vi "CRYGet CurveNames From Analysis.vi"(4 "Spectral Scaling":u16, 6 "Unit Info":T2={"Y unit In"="dB", "dB ref In"=1.0, "Y unit Out"="dB", "dB ref Out"=1.0, "Y unit Curve"="dB", "dB ref Curve"=1.0, "Y data  Curve"=0, "Y data Time"=0}, 8 "Harmonics array In":dbl[](array[numeric]) format="%.2f", 9 "Additional Option":T4(ring), 10 "Select Option":T5(ring), 11 "Algorithm":T6(ring)) -> (0 "Unit Info Out":T1, 1 "Display":T3={"display X"=TRUE, "display Y"=TRUE, "display Z"=TRUE}, 2 "Result":bool, 3 "Curves Name Out":string[](array[string]))   [LabVIEW 2013]
uses:
  Typedef Control/CRYUnit Info Cluster.ctl
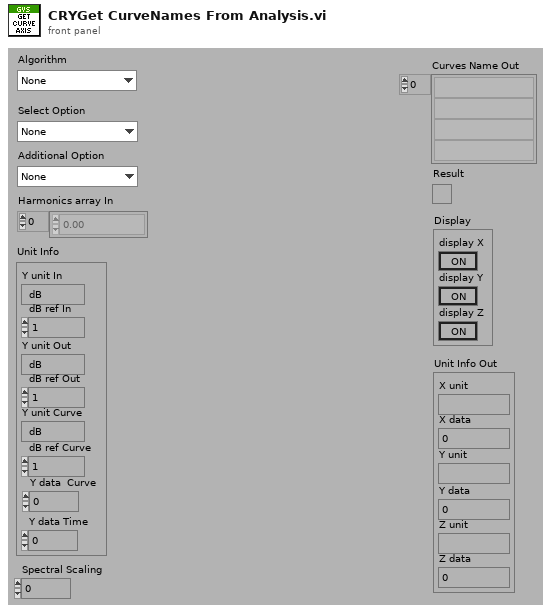
[diagram p1: front panel]
types:
  T1 = cluster{"X unit":string, "X data":u16, "Y unit":string, "Y data":u16, "Z unit":string, "Z data":u16}
  T2 = typedef "CRYUnit Info Cluster.ctl" = cluster{"Y unit In":string, "dB ref In":dbl, "Y unit Out":string, "dB ref Out":dbl, "Y unit Curve":string, "dB ref Curve":dbl, "Y data  Curve":u16, "Y data Time":u16}
  T3 = cluster{"display X":bool, "display Y":bool, "display Z":bool}
  T4 = enum16{"None", "Harmonic", "Intermodulation", "Difference", "DC Connect Measurement", "Complex", "Power"}
  T5 = enum16{"None", "Standard Error", "Confidence Limits", "Total Noise", "Harmonics meas.frq.", "Total Distortion", "THD", "THD Normalized", "THD + Noise", "Rub & Buzz", "Rub & Buzz Norm'd", "Total IM", "Total IMD", "Total IMD + Noise", "Total Diff", "Total DFD", "Total DFD + Noise", "Impulse Response", "Deconvolved Response", "Auto-Spectrum(Stimulus)", "Auto-Spectrum(Response)", "Frequency Response", "Cross-Spectrum", "Coherence", "Non-Coherence", "Signal-Noise Ratio", "Coherent Power", "Non-Coherent Power", "Non-Coherent Distortion", "Auto-Correlation(Stimulus)", "Auto-Correlation(Response)", "Cross-Correlation", "Impedence", "Auto Delay", "Time Envelop", "Loose Particle", "A(in Voltage)", "V(in Current)"}
  T6 = enum16{"None", "Broadband RMS", "Spectrum", "Hamonic Track", "Heterodyne", "Time Selective Response", "Multitone", "Transfer Function"}
  T7 = enum16{"None", "Standard Error", "Confidence Limits", "Total Noise", "Harmonics meas.frq.", "Total Distortion", "THD", "THD Normalized", "THD + Noise", "Rub & Buzz", "Rub & Buzz Norm'd", "Total IM", "Total IMD", "Total IMD + Noise", "Total Diff", "Total DFD", "Total DFD + Noise", "Impulse Response", "Deconvolved Response", "Auto-Spectrum(Stimulus)", "Auto-Spectrum(Response)", "Frequency Response", "Cross-Spectrum", "Coherence", "Non-Coherence", "Signal-Noise Ratio", "Coherent Power", "Non-Coherent Power", "Non-Coherent Distortion", "Auto-Correlation(Stimulus)", "Auto-Correlation(Response)", "Cross-Correlation", "Impedence", "Auto Delay", "Time Envelop", "Loose Particle"}
  T8 = cluster{"X unit":string, "X data":u16, "Y unit Curve":string, "Y data  Curve":u16, "Z unit":string, "X data":u16}
  T9 = cluster{"X unit":string, "X data":u16, string, "Y data  Curve":u16, "Z unit":string, "X data":u16}
  T10 = cluster{"X unit":string, "X data":u16, "Y unit Out":string, "Y data  Curve":u16, "Z unit":string, "X data":u16}
  T11 = cluster{"X unit":string, "X data":u16, "X unit":string, "X data":u16, "Z unit":string, "X data":u16}
  T12 = cluster{"X unit":string, "X data":u16, string, "Y data Time":u16, "Z unit":string, "X data":u16}
  T13 = cluster{"X unit":string, "X data":u16, "Y unit In":string, "Y data  Curve":u16, "Z unit":string, "X data":u16}
  T14 = cluster{"X unit":string, "X data":u16, "Z unit":string, "X data":u16, "Z unit":string, "X data":u16}
  T15 = cluster{"X unit":string, "X data":u16, "Y unit Out":string, "Y data Time":u16, "Z unit":string, "X data":u16}
  T16 = cluster{"X unit":string, "X data":u16, "Y unit In":string, "Y data Time":u16, "Z unit":string, "X data":u16}
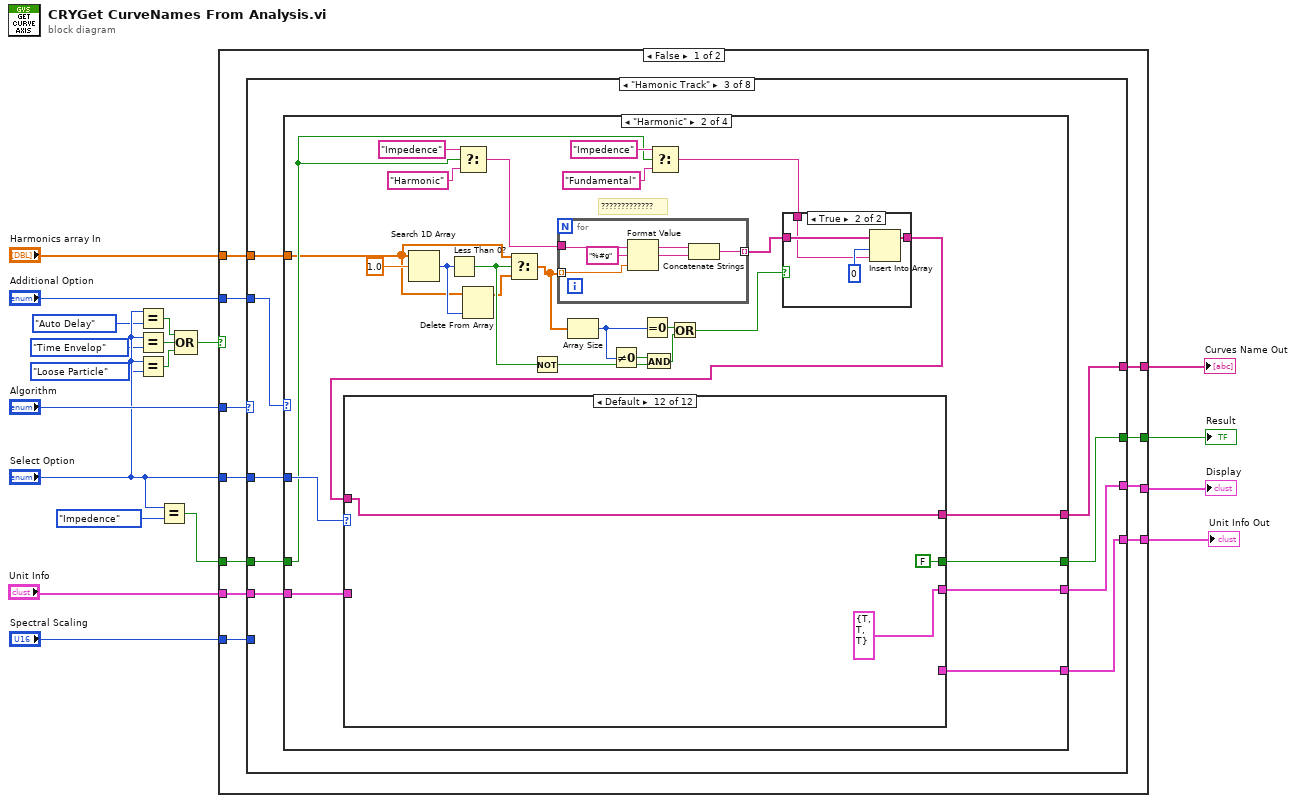
[diagram p0: block diagram]
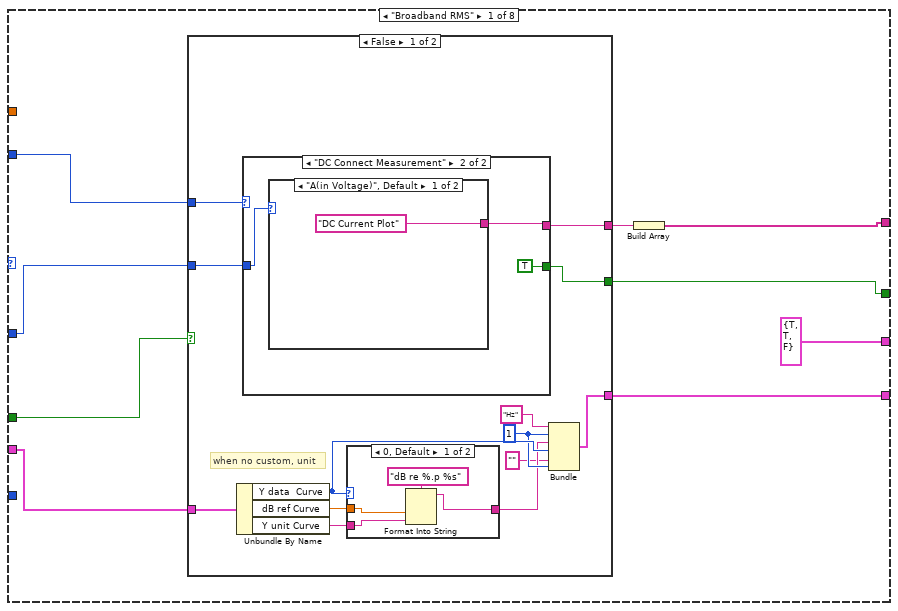
[diagram p2: hidden frame]
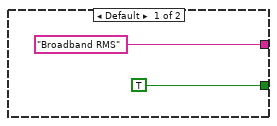
[diagram p4: hidden frame]
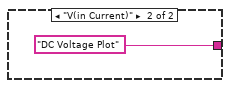
[diagram p5: hidden frame]
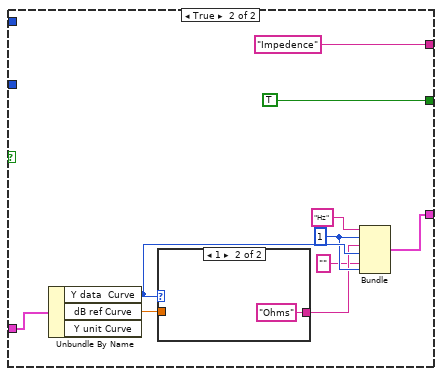
[diagram p6: hidden frame]
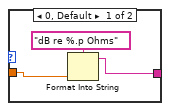
[diagram p7: hidden frame]
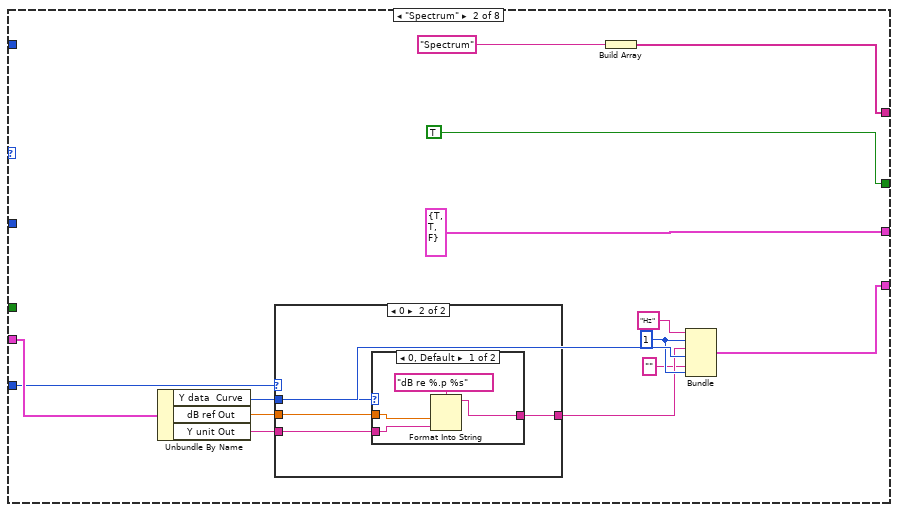
[diagram p8: hidden frame]
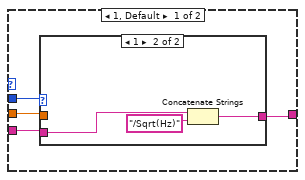
[diagram p9: hidden frame]
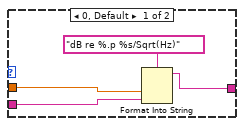
[diagram p10: hidden frame]
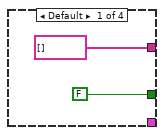
[diagram p12: hidden frame]
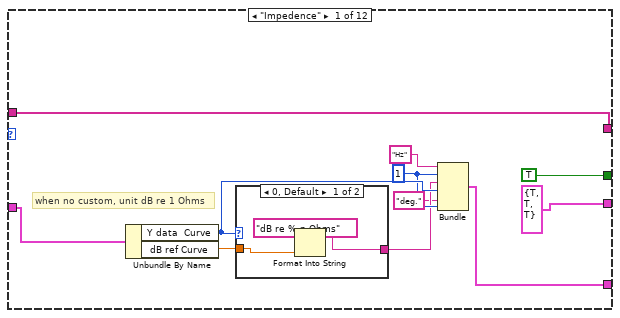
[diagram p14: hidden frame]
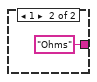
[diagram p15: hidden frame]
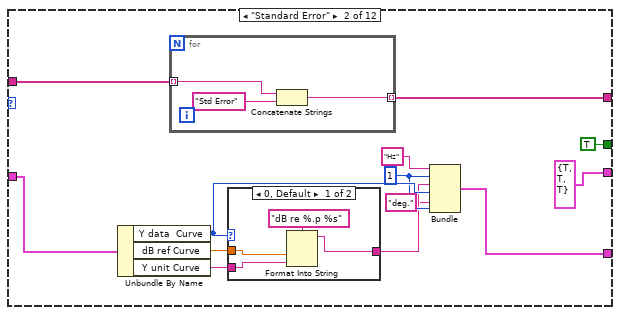
[diagram p16: hidden frame]
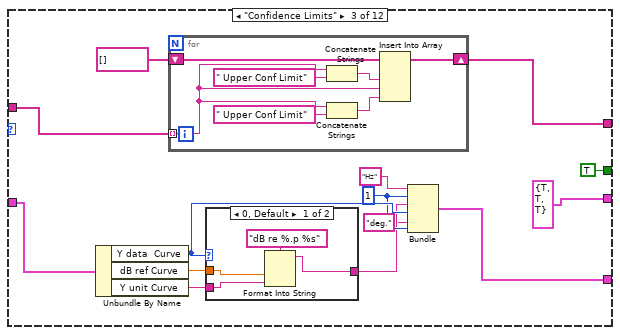
[diagram p18: hidden frame]
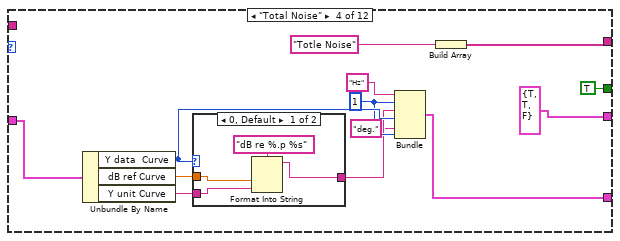
[diagram p20: hidden frame]
diagram:
  n1 = Equal?(x="Select Option", y=T7."Auto Delay") -> (x = y?=w14:bool)
  n2 = Equal?(x="Select Option", y=T7."Time Envelop") -> (x = y?=w13:bool)
  n3 = Equal?(x="Select Option", y=T7."Loose Particle") -> (x = y?=w12:bool)
  n4 = Equal?(x="Select Option", y=T7."Impedence") -> (x = y?=w10:bool)
  n5 = Compound Arithmetic op=OR(w14, w13, w12) -> (w11:bool)
  n6 = case shown="False" w11 {
    tunnel: "Algorithm" -> [w30 _]
    tunnel: "Select Option" -> [w29 w1352]
    tunnel: "Harmonics array In" -> [w28 _]
    tunnel: w10 -> [w27 _]
    tunnel: [w26 w1354] -> w17
    tunnel: [w25 w1353] -> w16
    tunnel: "Additional Option" -> [w24 _]
    tunnel: [w23 w1351] -> w4
    tunnel: "Unit Info" -> [w22 w1349]
    tunnel: [w21 w1350] -> w2
    tunnel: "Spectral Scaling" -> [w20 _]
    frame False {
      n7 = case shown="\"Hamonic Track\"" w30 {
        tunnel: w29 -> [w34 _ w118 _ w667 w777 w1012 _]
        tunnel: w28 -> [_ _ w121 _ w666 _ _ _]
        tunnel: w24 -> [w39 _ w120 _ _ w778 w1011 _]
        tunnel: w27 -> [w35 _ w119 w660 w668 w776 w1010 _]
        tunnel: [w37 w91 w117 w656 w665 w774 w1008 string[] []] -> w25
        tunnel: [w36 TRUE ("Result") w116 TRUE ("Result") w664 w773 w1007 FALSE ("Result")] -> w26
        tunnel: [T3 {"display X"=TRUE, "display Y"=TRUE, "display Z"=FALSE} T3 {"display X"=TRUE, "display Y"=TRUE, "display Z"=FALSE} w115 T3 {"display X"=TRUE, "display Y"=TRUE, "display Z"=TRUE} T3 {"display X"=TRUE, "display Y"=TRUE, "display Z"=TRUE} w772 w1006 _] -> w23
        tunnel: w22 -> [w31 w81 w113 _ w661 w771 w1004 _]
        tunnel: [w32 w80 w114 _ w662 w770 w1005 _] -> w21
        tunnel: w20 -> [_ w79 _ _ _ _ _ _]
        frame "Broadband RMS" {
          n8 = case shown="False" w35 {
            tunnel: [w51 "Impedence" ("string")] -> w38
            tunnel: w39 -> [w52 _]
            tunnel: [w50 TRUE ("Result")] -> w36
            tunnel: w34 -> [w49 _]
            tunnel: [w40 w65] -> w32
            tunnel: w31 -> [w41 w66]
            frame False {
              w45 = u16 1 ("X data")
              # "when no custom, unit"
              n9 = Unbundle By Name(w41) -> ("Y data  Curve"=w48:u16, "dB ref Curve"=w46:dbl, "Y unit Curve"=w47:string)
              n10 = case shown="\"DC Connect Measurement\"" w52 {
                tunnel: ["Broadband RMS" ("f") w62] -> w51
                tunnel: [TRUE ("Result") TRUE ("Result")] -> w50
                tunnel: w49 -> [_ w60]
                frame Default {
                }
                frame "DC Connect Measurement" {
                  n11 = case shown="\"A(in Voltage)\", Default" w60 {
                    tunnel: ["DC Current Plot" ("f") "DC Voltage Plot" ("f")] -> w62
                    frame "A(in Voltage)", Default {
                    }
                    frame "V(in Current)" {
                    }
                  }
                }
              }
              n12 = case shown="0, Default" w48 {
                tunnel: [w53 w57] -> w44
                tunnel: w46 -> [w54 _]
                tunnel: w47 -> [w55 w57]
                frame 0, Default {
                  n13 = Format Into String(format string="dB re %.p %s", w54, w55) -> (resulting string=w53:string)  [unwired: 2 in, 1 out]
                }
                frame 1 {
                }
              }
              n14 = Bundle("X unit"="Hz", "X data"=w45, "Y unit Curve"=w44, "Y data  Curve"=w48, "Z unit"="", "X data"=w45) -> (w40:T8)  [unwired: 1 in]
            }
            frame True {
              w70 = u16 1 ("X data")
              n15 = Unbundle By Name(w66) -> ("Y data  Curve"=w72:u16, "dB ref Curve"=w71:dbl)  [unwired: 1 out]
              n16 = case shown="1" w72 {
                tunnel: [w75 "Ohms"] -> w69
                tunnel: w71 -> [w76 _]
                frame 0, Default {
                  n17 = Format Into String(format string="dB re %.p Ohms", w76) -> (resulting string=w75:string)  [unwired: 2 in, 1 out]
                }
                frame 1 {
                }
              }
              n18 = Bundle("X unit"="Hz", "X data"=w70, w69, "Y data  Curve"=w72, "Z unit"="", "X data"=w70) -> (w65:T9)  [unwired: 1 in]
            }
          }
          n19 = Build Array(w38) -> (w37:string[])
        }
        frame "Spectrum" {
          w85 = u16 1 ("X data")
          n20 = Unbundle By Name(w81) -> ("Y data  Curve"=w88:u16, "dB ref Out"=w86:dbl, "Y unit Out"=w87:string)
          n21 = case shown="0" w79 {
            tunnel: w88 -> [w93 w107]
            tunnel: w87 -> [w95 w106]
            tunnel: w86 -> [w94 w105]
            tunnel: [w96 w104] -> w84
            frame 1, Default {
              n22 = case shown="1" w93 {
                tunnel: [w97 w101] -> w96
                tunnel: w94 -> [w98 _]
                tunnel: w95 -> [w99 w102]
                frame 0, Default {
                  n23 = Format Into String(format string="dB re %.p %s/Sqrt(Hz)", w98, w99) -> (resulting string=w97:string)  [unwired: 2 in, 1 out]
                }
                frame 1 {
                  n24 = Concatenate Strings(w102, "/Sqrt(Hz)" ("Y unit In")) -> (w101:string)
                }
              }
            }
            frame 0 {
              n25 = case shown="0, Default" w107 {
                tunnel: [w108 w112] -> w104
                tunnel: w105 -> [w109 _]
                tunnel: w106 -> [w110 w112]
                frame 0, Default {
                  n26 = Format Into String(format string="dB re %.p %s", w109, w110) -> (resulting string=w108:string)  [unwired: 2 in, 1 out]
                }
                frame 1 {
                }
              }
            }
          }
          n27 = Build Array("Spectrum" ("f")) -> (w91:string[])
          n28 = Bundle("X unit"="Hz", "X data"=w85, "Y unit Out"=w84, "Y data  Curve"=w88, "Z unit"="", "X data"=w85) -> (w80:T10)  [unwired: 1 in]
        }
        frame "Hamonic Track" {
          n29 = case shown="\"Harmonic\"" w120 {
            tunnel: w121 -> [_ w129 w342 w502]
            tunnel: w119 -> [_ w130 w341 w501]
            tunnel: w118 -> [_ w150 w340 w500]
            tunnel: [string[] [] w128 w338 w498] -> w117
            tunnel: [FALSE ("Result") w127 w337 w497] -> w116
            tunnel: [_ w126 w336 w494] -> w115
            tunnel: [_ w125 w335 w495] -> w114
            tunnel: w113 -> [_ w124 w334 w496]
            frame Default {
            }
            frame "Harmonic" {
              # "?????????????"
              n30 = Search 1D Array(1D array=w129, element=1.0) -> (index of element=w139:i32)  [unwired: 1 out]
              n31 = Less Than 0?(x=w139) -> (x < 0?=w146:bool)
              n32 = Select(t="Impedence", s=w130, f="Harmonic" ("string")) -> (s? t:f=w135:string)
              n33 = Delete From Array(array=w129, index=w139) -> (array with subset deleted=w140:dbl[])  [unwired: 1 in, 1 out]
              n34 = Select(t=w129, s=w146, f=w140) -> (s? t:f=w142:dbl[])
              n35 = Not(x=w146) -> (.not. x?=w147:bool)
              n36 = for {
                tunnel: w142 -> [w159] mode=indexing
                tunnel: [w157] -> w141 mode=indexing
                tunnel: w135 -> [w156]
                n37 = Format Value(format string="%#g", value (0)=w159) -> (output string=w158:string)  [unwired: 1 out]
                n38 = Concatenate Strings(w156, w158) -> (w157:string)
              }
              n39 = Array Size(array=w142) -> (size(s)=w144:i32)
              n40 = Not Equal To 0?(x=w144) -> (x != 0?=w145:bool)
              n41 = Equal To 0?(x=w144) -> (x = 0?=w143:bool)
              n42 = And(x=w145, y=w147) -> (x .and. y?=w148:bool)
              n43 = Select(t="Impedence", s=w130, f="Fundamental" ("string")) -> (s? t:f=w132:string)
              n44 = Or(x=w143, y=w148) -> (x .or. y?=w149:bool)
              n45 = case shown="True" w149 {
                tunnel: w141 -> [w151 w154]
                tunnel: [w151 w153] -> w131
                tunnel: w132 -> [_ w152]
                frame False {
                }
                frame True {
                  n46 = Insert Into Array(array=w154, index=0, new element=w152) -> (w153:string[])
                }
              }
              n47 = case shown="Default" w150 {
                tunnel: w131 -> [w171 w188 w209 _ w253 _ _ _ _ _ _ w332]
                tunnel: [w171 w187 w208 w234 w252 w279 w293 w302 w311 w320 w329 w332] -> w128
                tunnel: [TRUE ("Result") TRUE ("Result") TRUE ("Result") TRUE ("Result") TRUE ("Result") TRUE ("Result") TRUE ("Result") TRUE ("Result") TRUE ("Result") TRUE ("Result") TRUE ("Result") FALSE ("Result")] -> w127
                tunnel: [T3 {"display X"=TRUE, "display Y"=TRUE, "display Z"=TRUE} T3 {"display X"=TRUE, "display Y"=TRUE, "display Z"=TRUE} T3 {"display X"=TRUE, "display Y"=TRUE, "display Z"=TRUE} T3 {"display X"=TRUE, "display Y"=TRUE, "display Z"=FALSE} T3 {"display X"=TRUE, "display Y"=TRUE, "display Z"=TRUE} T3 {"display X"=TRUE, "display Y"=TRUE, "display Z"=TRUE} T3 {"display X"=TRUE, "display Y"=TRUE, "display Z"=FALSE} T3 {"display X"=TRUE, "display Y"=TRUE, "display Z"=FALSE} T3 {"display X"=TRUE, "display Y"=TRUE, "display Z"=FALSE} T3 {"display X"=TRUE, "display Y"=TRUE, "display Z"=FALSE} T3 {"display X"=TRUE, "display Y"=TRUE, "display Z"=FALSE} T3 {"display X"=TRUE, "display Y"=TRUE, "display Z"=TRUE}] -> w126
                tunnel: [w161 w177 w198 w224 w242 w269 w286 w295 w304 w313 w322 _] -> w125
                tunnel: w124 -> [w163 w178 w199 w223 w243 w268 _ _ _ _ _ _]
                frame "Impedence" {
                  w166 = u16 1 ("X data")
                  # "when no custom, unit dB re 1 Ohms"
                  n48 = Unbundle By Name(w163) -> ("Y data  Curve"=w168:u16, "dB ref Curve"=w167:dbl)
                  n49 = case shown="0, Default" w168 {
                    tunnel: [w172 "Ohms"] -> w165
                    tunnel: w167 -> [w173 _]
                    frame 0, Default {
                      n50 = Format Into String(format string="dB re %.p Ohms", w173) -> (resulting string=w172:string)  [unwired: 2 in, 1 out]
                    }
                    frame 1 {
                    }
                  }
                  n51 = Bundle("X unit"="Hz", "X data"=w166, w165, "Y data  Curve"=w168, "Z unit"="deg.", "X data"=w166) -> (w161:T9)  [unwired: 1 in]
                }
                frame "Standard Error" {
                  w182 = u16 1 ("X data")
                  n52 = Unbundle By Name(w178) -> ("Y data  Curve"=w185:u16, "dB ref Curve"=w183:dbl, "Y unit Curve"=w184:string)
                  n53 = for {
                    tunnel: w188 -> [w196] mode=indexing
                    tunnel: [w194] -> w187 mode=indexing
                    n54 = Concatenate Strings(w196, "Std Error" ("string")) -> (w194:string)
                  }
                  n55 = case shown="0, Default" w185 {
                    tunnel: [w189 w193] -> w181
                    tunnel: w183 -> [w190 _]
                    tunnel: w184 -> [w191 w193]
                    frame 0, Default {
                      n56 = Format Into String(format string="dB re %.p %s", w190, w191) -> (resulting string=w189:string)  [unwired: 2 in, 1 out]
                    }
                    frame 1 {
                    }
                  }
                  n57 = Bundle("X unit"="Hz", "X data"=w182, "Y unit Curve"=w181, "Y data  Curve"=w185, "Z unit"="deg.", "X data"=w182) -> (w177:T8)  [unwired: 1 in]
                }
                frame "Confidence Limits" {
                  w203 = u16 1 ("X data")
                  n58 = Unbundle By Name(w199) -> ("Y data  Curve"=w206:u16, "dB ref Curve"=w204:dbl, "Y unit Curve"=w205:string)
                  n59 = for {
                    shift-right: [w216] -> w208
                    shift-left: string[] [] -> [w217]
                    tunnel: w209 -> [w218] mode=indexing
                    n60 = Concatenate Strings(w218, " Upper Conf Limit" ("string")) -> (w220:string)
                    n61 = Concatenate Strings(w218, " Upper Conf Limit" ("string")) -> (w221:string)
                    n62 = Insert Into Array(array=w217, new element #1=w220, new element #2=w218, new element #3=w221) -> (w216:string[])  [unwired: 1 in]
                  }
                  n63 = case shown="0, Default" w206 {
                    tunnel: [w211 w215] -> w202
                    tunnel: w204 -> [w212 _]
                    tunnel: w205 -> [w213 w215]
                    frame 0, Default {
                      n64 = Format Into String(format string="dB re %.p %s", w212, w213) -> (resulting string=w211:string)  [unwired: 2 in, 1 out]
                    }
                    frame 1 {
                    }
                  }
                  n65 = Bundle("X unit"="Hz", "X data"=w203, "Y unit Curve"=w202, "Y data  Curve"=w206, "Z unit"="deg.", "X data"=w203) -> (w198:T8)  [unwired: 1 in]
                }
                frame "Total Noise" {
                  w229 = u16 1 ("X data")
                  n66 = Unbundle By Name(w223) -> ("Y data  Curve"=w232:u16, "dB ref Curve"=w230:dbl, "Y unit Curve"=w231:string)
                  n67 = case shown="0, Default" w232 {
                    tunnel: [w236 w240] -> w228
                    tunnel: w230 -> [w237 _]
                    tunnel: w231 -> [w238 w240]
                    frame 0, Default {
                      n68 = Format Into String(format string="dB re %.p %s", w237, w238) -> (resulting string=w236:string)  [unwired: 2 in, 1 out]
                    }
                    frame 1 {
                    }
                  }
                  n69 = Bundle("X unit"="Hz", "X data"=w229, "Y unit Curve"=w228, "Y data  Curve"=w232, "Z unit"="deg.", "X data"=w229) -> (w224:T8)  [unwired: 1 in]
                  n70 = Build Array("Totle Noise" ("new element/subarray")) -> (w234:string[])
                }
                frame "Harmonics meas.frq." {
                  w247 = u16 1 ("X data")
                  n71 = Unbundle By Name(w243) -> ("Y data  Curve"=w250:u16, "dB ref Curve"=w248:dbl, "Y unit Curve"=w249:string)
                  n72 = Array Size(array=w253) -> (size(s)=w254:i32)
                  n73 = Decrement(x=w254) -> (x-1=w255:i32)
                  n74 = for {
                    N: w255 -> [_]
                    tunnel: w253 -> [w267]
                    tunnel: [w262] -> w256 mode=indexing
                    i -> [w266]
                    n75 = Increment(x=w266) -> (x+1=w265:i32)
                    n76 = Index Array(array=w267, index=w265) -> (element=w264:string)
                    n77 = Concatenate Strings(w264, "at meas. freq." ("string")) -> (w262:string)
                  }
                  n78 = case shown="0, Default" w250 {
                    tunnel: [w257 w261] -> w246
                    tunnel: w248 -> [w258 _]
                    tunnel: w249 -> [w259 w261]
                    frame 0, Default {
                      n79 = Format Into String(format string="dB re %.p %s", w258, w259) -> (resulting string=w257:string)  [unwired: 2 in, 1 out]
                    }
                    frame 1 {
                    }
                  }
                  n80 = Bundle("X unit"="Hz", "X data"=w247, "Y unit Curve"=w246, "Y data  Curve"=w250, "Z unit"="deg.", "X data"=w247) -> (w242:T8)  [unwired: 1 in]
                  n81 = Insert Into Array(array=w253, new element=w256) -> (w252:string[])  [unwired: 1 in]
                }
                frame "Total Distortion" {
                  w274 = u16 1 ("X data")
                  n82 = Unbundle By Name(w268) -> ("Y data  Curve"=w277:u16, "dB ref Curve"=w275:dbl, "Y unit Curve"=w276:string)
                  n83 = case shown="0, Default" w277 {
                    tunnel: [w281 w285] -> w273
                    tunnel: w275 -> [w282 _]
                    tunnel: w276 -> [w283 w285]
                    frame 0, Default {
                      n84 = Format Into String(format string="dB re %.p %s", w282, w283) -> (resulting string=w281:string)  [unwired: 2 in, 1 out]
                    }
                    frame 1 {
                    }
                  }
                  n85 = Build Array("Total Distortion" ("new element/subarray")) -> (w279:string[])
                  n86 = Bundle("X unit"="Hz", "X data"=w274, "Y unit Curve"=w273, "Y data  Curve"=w277, "Z unit"="deg.", "X data"=w274) -> (w269:T8)  [unwired: 1 in]
                }
                frame "THD" {
                  w290 = u16 1 ("X data")
                  n87 = Bundle("X unit"="Hz", "X data"=w290, "X unit"="%", "X data"=w290, "Z unit"="", "X data"=w290) -> (w286:T11)  [unwired: 1 in]
                  n88 = Build Array("THD" ("new element/subarray")) -> (w293:string[])
                }
                frame "THD Normalized" {
                  w299 = u16 1 ("X data")
                  n89 = Build Array("THD Normalized" ("new element/subarray")) -> (w302:string[])
                  n90 = Bundle("X unit"="Hz", "X data"=w299, "X unit"="%", "X data"=w299, "Z unit"="", "X data"=w299) -> (w295:T11)  [unwired: 1 in]
                }
                frame "THD + Noise" {
                  w308 = u16 1 ("X data")
                  n91 = Build Array("THD+N" ("new element/subarray")) -> (w311:string[])
                  n92 = Bundle("X unit"="Hz", "X data"=w308, "X unit"="%", "X data"=w308, "Z unit"="", "X data"=w308) -> (w304:T11)  [unwired: 1 in]
                }
                frame "Rub & Buzz" {
                  w317 = u16 1 ("X data")
                  n93 = Build Array("Rub & Buzz" ("new element/subarray")) -> (w320:string[])
                  n94 = Bundle("X unit"="Hz", "X data"=w317, "X unit"="%", "X data"=w317, "Z unit"="", "X data"=w317) -> (w313:T11)  [unwired: 1 in]
                }
                frame "Rub & Buzz Norm'd" {
                  w326 = u16 1 ("X data")
                  n95 = Build Array("Rub & Buzz Normalized" ("new element/subarray")) -> (w329:string[])
                  n96 = Bundle("X unit"="Hz", "X data"=w326, "X unit"="%", "X data"=w326, "Z unit"="", "X data"=w326) -> (w322:T11)  [unwired: 1 in]
                }
                frame Default {
                }
              }
            }
            frame "Intermodulation" {
              n97 = Search 1D Array(1D array=w342, element=1.0) -> (index of element=w347:i32)  [unwired: 1 out]
              n98 = Less Than 0?(x=w347) -> (x < 0?=w354:bool)
              n99 = Select(t="Impedence", s=w341, f="IM" ("string")) -> (s? t:f=w343:string)
              n100 = Delete From Array(array=w342, index=w347) -> (array with subset deleted=w348:dbl[])  [unwired: 1 in, 1 out]
              n101 = Select(t=w342, s=w354, f=w348) -> (s? t:f=w350:dbl[])
              n102 = Not(x=w354) -> (.not. x?=w355:bool)
              n103 = for {
                tunnel: w350 -> [w492] mode=indexing
                tunnel: [w490] -> w349 mode=indexing
                tunnel: w343 -> [w489]
                n104 = Format Value(format string="%#g", value (0)=w492) -> (output string=w491:string)  [unwired: 1 out]
                n105 = Concatenate Strings(w489, w491) -> (w490:string)
              }
              n106 = Array Size(array=w350) -> (size(s)=w352:i32)
              n107 = Not Equal To 0?(x=w352) -> (x != 0?=w353:bool)
              n108 = Equal To 0?(x=w352) -> (x = 0?=w351:bool)
              n109 = And(x=w353, y=w355) -> (x .and. y?=w356:bool)
              n110 = Or(x=w351, y=w356) -> (x .or. y?=w357:bool)
              n111 = case shown="True" w357 {
                tunnel: w349 -> [w476 w479]
                tunnel: [w476 w478] -> w339
                tunnel: w341 -> [_ w477]
                frame False {
                }
                frame True {
                  n112 = case shown="True" w477 {
                    tunnel: w479 -> [w484 w487]
                    tunnel: [w480 w486] -> w478
                    frame False {
                      n113 = Insert Into Array(array=w484, index=0, new element #1="IM Fundamental" ("new element/subarray"), new element #2="IM Fixed Tone" ("new element/subarray")) -> (w480:string[])
                    }
                    frame True {
                      n114 = Insert Into Array(array=w487, index=0, new element="Impedence" ("new element/subarray")) -> (w486:string[])
                    }
                  }
                }
              }
              n115 = case shown="\"Impedence\"" w340 {
                tunnel: w339 -> [w368 w385 w406 _ _ _ _ _]
                tunnel: [w368 w384 w405 w431 w449 w463 w472 string[] []] -> w338
                tunnel: [TRUE ("Result") TRUE ("Result") TRUE ("Result") TRUE ("Result") TRUE ("Result") TRUE ("Result") TRUE ("Result") FALSE ("Result")] -> w337
                tunnel: [T3 {"display X"=TRUE, "display Y"=TRUE, "display Z"=TRUE} T3 {"display X"=TRUE, "display Y"=TRUE, "display Z"=TRUE} T3 {"display X"=TRUE, "display Y"=TRUE, "display Z"=TRUE} T3 {"display X"=TRUE, "display Y"=TRUE, "display Z"=FALSE} T3 {"display X"=TRUE, "display Y"=TRUE, "display Z"=TRUE} T3 {"display X"=TRUE, "display Y"=TRUE, "display Z"=FALSE} T3 {"display X"=TRUE, "display Y"=TRUE, "display Z"=FALSE} _] -> w336
                tunnel: [w359 w374 w395 w421 w439 w457 w466 _] -> w335
                tunnel: w334 -> [w358 w373 w394 w422 w440 _ _ _]
                frame "Impedence" {
                  w364 = u16 1 ("X data")
                  # "when no custom, unit dB re 1 Ohms"
                  n116 = Unbundle By Name(w358) -> ("Y data  Curve"=w366:u16, "dB ref Curve"=w365:dbl)
                  n117 = case shown="0, Default" w366 {
                    tunnel: [w369 "Ohms"] -> w363
                    tunnel: w365 -> [w370 _]
                    frame 0, Default {
                      n118 = Format Into String(format string="dB re %.p Ohms", w370) -> (resulting string=w369:string)  [unwired: 2 in, 1 out]
                    }
                    frame 1 {
                    }
                  }
                  n119 = Bundle("X unit"="Hz", "X data"=w364, w363, "Y data  Curve"=w366, "Z unit"="deg.", "X data"=w364) -> (w359:T9)  [unwired: 1 in]
                }
                frame "Standard Error" {
                  w379 = u16 1 ("X data")
                  n120 = Unbundle By Name(w373) -> ("Y data  Curve"=w376:u16, "dB ref Curve"=w378:dbl, "Y unit Curve"=w377:string)
                  n121 = for {
                    tunnel: w385 -> [w392] mode=indexing
                    tunnel: [w391] -> w384 mode=indexing
                    n122 = Concatenate Strings(w392, "Std Error" ("string")) -> (w391:string)
                  }
                  n123 = case shown="0, Default" w376 {
                    tunnel: [w386 w390] -> w380
                    tunnel: w378 -> [w387 _]
                    tunnel: w377 -> [w388 w390]
                    frame 0, Default {
                      n124 = Format Into String(format string="dB re %.p %s", w387, w388) -> (resulting string=w386:string)  [unwired: 2 in, 1 out]
                    }
                    frame 1 {
                    }
                  }
                  n125 = Bundle("X unit"="Hz", "X data"=w379, "Y unit Curve"=w380, "Y data  Curve"=w376, "Z unit"="deg.", "X data"=w379) -> (w374:T8)  [unwired: 1 in]
                }
                frame "Confidence Limits" {
                  w400 = u16 1 ("X data")
                  n126 = Unbundle By Name(w394) -> ("Y data  Curve"=w397:u16, "dB ref Curve"=w399:dbl, "Y unit Curve"=w398:string)
                  n127 = for {
                    shift-right: [w414] -> w405
                    shift-left: string[] [] -> [w415]
                    tunnel: w406 -> [w413] mode=indexing
                    n128 = Concatenate Strings(w413, " Upper Conf Limit" ("string")) -> (w417:string)
                    n129 = Concatenate Strings(w413, " Upper Conf Limit" ("string")) -> (w418:string)
                    n130 = Insert Into Array(array=w415, new element #1=w417, new element #2=w413, new element #3=w418) -> (w414:string[])  [unwired: 1 in]
                  }
                  n131 = case shown="0, Default" w397 {
                    tunnel: [w408 w412] -> w401
                    tunnel: w399 -> [w409 _]
                    tunnel: w398 -> [w410 w412]
                    frame 0, Default {
                      n132 = Format Into String(format string="dB re %.p %s", w409, w410) -> (resulting string=w408:string)  [unwired: 2 in, 1 out]
                    }
                    frame 1 {
                    }
                  }
                  n133 = Bundle("X unit"="Hz", "X data"=w400, "Y unit Curve"=w401, "Y data  Curve"=w397, "Z unit"="deg.", "X data"=w400) -> (w395:T8)  [unwired: 1 in]
                }
                frame "Total Noise" {
                  w426 = u16 1 ("X data")
                  n134 = Unbundle By Name(w422) -> ("Y data  Curve"=w423:u16, "dB ref Curve"=w425:dbl, "Y unit Curve"=w424:string)
                  n135 = case shown="0, Default" w423 {
                    tunnel: [w433 w437] -> w427
                    tunnel: w425 -> [w434 _]
                    tunnel: w424 -> [w435 w437]
                    frame 0, Default {
                      n136 = Format Into String(format string="dB re %.p %s", w434, w435) -> (resulting string=w433:string)  [unwired: 2 in, 1 out]
                    }
                    frame 1 {
                    }
                  }
                  n137 = Build Array("Totle Noise" ("new element/subarray")) -> (w431:string[])
                  n138 = Bundle("X unit"="Hz", "X data"=w426, "Y unit Curve"=w427, "Y data  Curve"=w423, "Z unit"="deg.", "X data"=w426) -> (w421:T8)  [unwired: 1 in]
                }
                frame "Total IM" {
                  w444 = u16 1 ("X data")
                  n139 = Unbundle By Name(w440) -> ("Y data  Curve"=w441:u16, "dB ref Curve"=w443:dbl, "Y unit Curve"=w442:string)
                  n140 = case shown="0, Default" w441 {
                    tunnel: [w451 w455] -> w445
                    tunnel: w443 -> [w452 _]
                    tunnel: w442 -> [w453 w455]
                    frame 0, Default {
                      n141 = Format Into String(format string="dB re %.p %s", w452, w453) -> (resulting string=w451:string)  [unwired: 2 in, 1 out]
                    }
                    frame 1 {
                    }
                  }
                  n142 = Build Array("Total IM" ("new element/subarray")) -> (w449:string[])
                  n143 = Bundle("X unit"="Hz", "X data"=w444, "Y unit Curve"=w445, "Y data  Curve"=w441, "Z unit"="deg.", "X data"=w444) -> (w439:T8)  [unwired: 1 in]
                }
                frame "Total IMD" {
                  w458 = u16 1 ("X data")
                  n144 = Build Array("Total IMD" ("new element/subarray")) -> (w463:string[])
                  n145 = Bundle("X unit"="Hz", "X data"=w458, "X unit"="%", "X data"=w458, "Z unit"="", "X data"=w458) -> (w457:T11)  [unwired: 1 in]
                }
                frame "Total IMD + Noise" {
                  w470 = u16 1 ("X data")
                  n146 = Build Array("Total IMD + N" ("new element/subarray")) -> (w472:string[])
                  n147 = Bundle("X unit"="Hz", "X data"=w470, "X unit"="%", "X data"=w470, "Z unit"="", "X data"=w470) -> (w466:T11)  [unwired: 1 in]
                }
                frame Default {
                }
              }
            }
            frame "Difference" {
              n148 = Search 1D Array(1D array=w502, element=1.0) -> (index of element=w507:i32)  [unwired: 1 out]
              n149 = Less Than 0?(x=w507) -> (x < 0?=w514:bool)
              n150 = Select(t="Impedence", s=w501, f="Diff" ("string")) -> (s? t:f=w503:string)
              n151 = Delete From Array(array=w502, index=w507) -> (array with subset deleted=w508:dbl[])  [unwired: 1 in, 1 out]
              n152 = Select(t=w502, s=w514, f=w508) -> (s? t:f=w510:dbl[])
              n153 = Not(x=w514) -> (.not. x?=w515:bool)
              n154 = for {
                tunnel: w510 -> [w652] mode=indexing
                tunnel: [w650] -> w509 mode=indexing
                tunnel: w503 -> [w649]
                n155 = Format Value(format string="%#g", value (0)=w652) -> (output string=w651:string)  [unwired: 1 out]
                n156 = Concatenate Strings(w649, w651) -> (w650:string)
              }
              n157 = Array Size(array=w510) -> (size(s)=w512:i32)
              n158 = Not Equal To 0?(x=w512) -> (x != 0?=w513:bool)
              n159 = Equal To 0?(x=w512) -> (x = 0?=w511:bool)
              n160 = And(x=w513, y=w515) -> (x .and. y?=w516:bool)
              n161 = Or(x=w511, y=w516) -> (x .or. y?=w517:bool)
              n162 = case shown="True" w517 {
                tunnel: w509 -> [w636 w639]
                tunnel: [w636 w638] -> w499
                tunnel: w501 -> [_ w637]
                frame False {
                }
                frame True {
                  n163 = case shown="False" w637 {
                    tunnel: w639 -> [w644 w647]
                    tunnel: [w640 w646] -> w638
                    frame False {
                      n164 = Insert Into Array(array=w644, index=0, new element #1="Diff Upper Fundamental" ("new element/subarray"), new element #2="Diff Lower Fundamental" ("new element/subarray")) -> (w640:string[])
                    }
                    frame True {
                      n165 = Insert Into Array(array=w647, index=0, new element="Impedence" ("new element/subarray")) -> (w646:string[])
                    }
                  }
                }
              }
              n166 = case shown="Default" w500 {
                tunnel: w499 -> [w528 w545 w565 _ _ _ _ _]
                tunnel: [w528 w544 w566 w591 w609 w623 w632 string[] []] -> w498
                tunnel: [TRUE ("Result") TRUE ("Result") TRUE ("Result") TRUE ("Result") TRUE ("Result") TRUE ("Result") TRUE ("Result") FALSE ("Result")] -> w497
                tunnel: w496 -> [w520 w535 w556 w583 w600 _ _ _]
                tunnel: [w519 w534 w555 w582 w599 w617 w625 _] -> w495
                tunnel: [T3 {"display X"=TRUE, "display Y"=TRUE, "display Z"=TRUE} T3 {"display X"=TRUE, "display Y"=TRUE, "display Z"=TRUE} T3 {"display X"=TRUE, "display Y"=TRUE, "display Z"=TRUE} T3 {"display X"=TRUE, "display Y"=TRUE, "display Z"=FALSE} T3 {"display X"=TRUE, "display Y"=TRUE, "display Z"=TRUE} T3 {"display X"=TRUE, "display Y"=TRUE, "display Z"=FALSE} T3 {"display X"=TRUE, "display Y"=TRUE, "display Z"=FALSE} _] -> w494
                frame "Impedence" {
                  w523 = u16 1 ("X data")
                  # "when no custom, unit dB re 1 Ohms"
                  n167 = Unbundle By Name(w520) -> ("Y data  Curve"=w521:u16, "dB ref Curve"=w522:dbl)
                  n168 = case shown="0, Default" w521 {
                    tunnel: [w529 "Ohms"] -> w524
                    tunnel: w522 -> [w530 _]
                    frame 0, Default {
                      n169 = Format Into String(format string="dB re %.p Ohms", w530) -> (resulting string=w529:string)  [unwired: 2 in, 1 out]
                    }
                    frame 1 {
                    }
                  }
                  n170 = Bundle("X unit"="Hz", "X data"=w523, w524, "Y data  Curve"=w521, "Z unit"="deg.", "X data"=w523) -> (w519:T9)  [unwired: 1 in]
                }
                frame "Standard Error" {
                  w539 = u16 1 ("X data")
                  n171 = Unbundle By Name(w535) -> ("Y data  Curve"=w536:u16, "dB ref Curve"=w538:dbl, "Y unit Curve"=w537:string)
                  n172 = case shown="0, Default" w536 {
                    tunnel: [w546 w550] -> w540
                    tunnel: w538 -> [w547 _]
                    tunnel: w537 -> [w548 w550]
                    frame 0, Default {
                      n173 = Format Into String(format string="dB re %.p %s", w547, w548) -> (resulting string=w546:string)  [unwired: 2 in, 1 out]
                    }
                    frame 1 {
                    }
                  }
                  n174 = for {
                    tunnel: w545 -> [w553] mode=indexing
                    tunnel: [w552] -> w544 mode=indexing
                    n175 = Concatenate Strings(w553, "Std Error" ("string")) -> (w552:string)
                  }
                  n176 = Bundle("X unit"="Hz", "X data"=w539, "Y unit Curve"=w540, "Y data  Curve"=w536, "Z unit"="deg.", "X data"=w539) -> (w534:T8)  [unwired: 1 in]
                }
                frame "Confidence Limits" {
                  w560 = u16 1 ("X data")
                  n177 = Unbundle By Name(w556) -> ("Y data  Curve"=w557:u16, "dB ref Curve"=w559:dbl, "Y unit Curve"=w558:string)
                  n178 = for {
                    shift-right: [w574] -> w566
                    shift-left: string[] [] -> [w575]
                    tunnel: w565 -> [w573] mode=indexing
                    n179 = Concatenate Strings(w573, " Upper Conf Limit" ("string")) -> (w577:string)
                    n180 = Concatenate Strings(w573, " Upper Conf Limit" ("string")) -> (w578:string)
                    n181 = Insert Into Array(array=w575, new element #1=w577, new element #2=w573, new element #3=w578) -> (w574:string[])  [unwired: 1 in]
                  }
                  n182 = case shown="0, Default" w557 {
                    tunnel: [w568 w572] -> w561
                    tunnel: w559 -> [w569 _]
                    tunnel: w558 -> [w570 w572]
                    frame 0, Default {
                      n183 = Format Into String(format string="dB re %.p %s", w569, w570) -> (resulting string=w568:string)  [unwired: 2 in, 1 out]
                    }
                    frame 1 {
                    }
                  }
                  n184 = Bundle("X unit"="Hz", "X data"=w560, "Y unit Curve"=w561, "Y data  Curve"=w557, "Z unit"="deg.", "X data"=w560) -> (w555:T8)  [unwired: 1 in]
                }
                frame "Total Noise" {
                  w587 = u16 1 ("X data")
                  n185 = Unbundle By Name(w583) -> ("Y data  Curve"=w584:u16, "dB ref Curve"=w586:dbl, "Y unit Curve"=w585:string)
                  n186 = case shown="0, Default" w584 {
                    tunnel: [w593 w597] -> w588
                    tunnel: w586 -> [w594 _]
                    tunnel: w585 -> [w595 w597]
                    frame 0, Default {
                      n187 = Format Into String(format string="dB re %.p %s", w594, w595) -> (resulting string=w593:string)  [unwired: 2 in, 1 out]
                    }
                    frame 1 {
                    }
                  }
                  n188 = Build Array("Totle Noise" ("new element/subarray")) -> (w591:string[])
                  n189 = Bundle("X unit"="Hz", "X data"=w587, "Y unit Curve"=w588, "Y data  Curve"=w584, "Z unit"="deg.", "X data"=w587) -> (w582:T8)  [unwired: 1 in]
                }
                frame "Total Diff" {
                  w604 = u16 1 ("X data")
                  n190 = Unbundle By Name(w600) -> ("Y data  Curve"=w601:u16, "dB ref Curve"=w603:dbl, "Y unit Curve"=w602:string)
                  n191 = case shown="0, Default" w601 {
                    tunnel: [w611 w615] -> w605
                    tunnel: w603 -> [w612 _]
                    tunnel: w602 -> [w613 w615]
                    frame 0, Default {
                      n192 = Format Into String(format string="dB re %.p %s", w612, w613) -> (resulting string=w611:string)  [unwired: 2 in, 1 out]
                    }
                    frame 1 {
                    }
                  }
                  n193 = Bundle("X unit"="Hz", "X data"=w604, "Y unit Curve"=w605, "Y data  Curve"=w601, "Z unit"="deg.", "X data"=w604) -> (w599:T8)  [unwired: 1 in]
                  n194 = Build Array("Total Diff" ("new element/subarray")) -> (w609:string[])
                }
                frame "Total DFD" {
                  w618 = u16 1 ("X data")
                  n195 = Build Array("Total DFD" ("new element/subarray")) -> (w623:string[])
                  n196 = Bundle("X unit"="Hz", "X data"=w618, "X unit"="%", "X data"=w618, "Z unit"="", "X data"=w618) -> (w617:T11)  [unwired: 1 in]
                }
                frame "Total DFD + Noise" {
                  w627 = u16 1 ("X data")
                  n197 = Build Array("Total DFD + N" ("new element/subarray")) -> (w632:string[])
                  n198 = Bundle("X unit"="Hz", "X data"=w627, "X unit"="%", "X data"=w627, "Z unit"="", "X data"=w627) -> (w625:T11)  [unwired: 1 in]
                }
                frame Default {
                }
              }
            }
          }
        }
        frame "Heterodyne" {
          n199 = Select(t="Impedence" ("f"), s=w660, f="Fundamental") -> (s? t:f=w657:string)
          n200 = Build Array(w657) -> (w656:string[])
        }
        frame "Time Selective Response" {
          n201 = Search 1D Array(1D array=w666, element=1.0) -> (index of element=w677:i32)  [unwired: 1 out]
          n202 = Less Than 0?(x=w677) -> (x < 0?=w684:bool)
          n203 = Select(t="Impedence", s=w668, f="Harmonic" ("string")) -> (s? t:f=w673:string)
          n204 = Delete From Array(array=w666, index=w677) -> (array with subset deleted=w678:dbl[])  [unwired: 1 in, 1 out]
          n205 = Select(t=w666, s=w684, f=w678) -> (s? t:f=w680:dbl[])
          n206 = Not(x=w684) -> (.not. x?=w685:bool)
          n207 = for {
            tunnel: w680 -> [w696] mode=indexing
            tunnel: [w694] -> w679 mode=indexing
            tunnel: w673 -> [w693]
            n208 = Format Value(format string="%.1f", value (0)=w696) -> (output string=w695:string)  [unwired: 1 out]
            n209 = Concatenate Strings(w693, w695) -> (w694:string)
          }
          n210 = Array Size(array=w680) -> (size(s)=w682:i32)
          n211 = Not Equal To 0?(x=w682) -> (x != 0?=w683:bool)
          n212 = Equal To 0?(x=w682) -> (x = 0?=w681:bool)
          n213 = And(x=w683, y=w685) -> (x .and. y?=w686:bool)
          n214 = Select(t="Impedence", s=w668, f="Fundamental" ("string")) -> (s? t:f=w670:string)
          n215 = Or(x=w681, y=w686) -> (x .or. y?=w687:bool)
          n216 = case shown="True" w687 {
            tunnel: w679 -> [w688 w691]
            tunnel: [w688 w690] -> w669
            tunnel: w670 -> [_ w689]
            frame False {
            }
            frame True {
              n217 = Insert Into Array(array=w691, index=0, new element=w689) -> (w690:string[])
            }
          }
          n218 = case shown="\"Deconvolved Response\"" w667 {
            tunnel: w669 -> [w699 w702 _ _ _ _ _ _ _ _ _]
            tunnel: [w699 w701 w713 w716 w719 w722 w725 w728 w740 w759 string[] []] -> w665
            tunnel: [TRUE ("Result") TRUE ("Result") TRUE ("Result") TRUE ("Result") TRUE ("Result") TRUE ("Result") TRUE ("Result") TRUE ("Result") TRUE ("Result") TRUE ("Result") FALSE ("Result")] -> w664
            tunnel: [_ _ _ _ _ _ _ _ w730 w750 _] -> w662
            tunnel: w661 -> [_ _ _ _ _ _ _ _ w731 w749 _]
            frame "None", "Impedence" {
            }
            frame "Harmonics meas.frq." {
              n219 = Array Size(array=w702) -> (size(s)=w703:i32)
              n220 = Decrement(x=w703) -> (x-1=w704:i32)
              n221 = for {
                N: w704 -> [_]
                tunnel: w702 -> [w711]
                tunnel: [w706] -> w705 mode=indexing
                i -> [w710]
                n222 = Increment(x=w710) -> (x+1=w709:i32)
                n223 = Index Array(array=w711, index=w709) -> (element=w708:string)
                n224 = Concatenate Strings(w708, "at meas. freq." ("string")) -> (w706:string)
              }
              n225 = Insert Into Array(array=w702, new element=w705) -> (w701:string[])  [unwired: 1 in]
            }
            frame "Total Distortion" {
              n226 = Build Array("Total Distortion" ("new element/subarray")) -> (w713:string[])
            }
            frame "THD" {
              n227 = Build Array("THD" ("new element/subarray")) -> (w716:string[])
            }
            frame "THD Normalized" {
              n228 = Build Array("THD Normalized" ("new element/subarray")) -> (w719:string[])
            }
            frame "THD + Noise" {
              n229 = Build Array("THD+N" ("new element/subarray")) -> (w722:string[])
            }
            frame "Rub & Buzz" {
              n230 = Build Array("Rub & Buzz" ("new element/subarray")) -> (w725:string[])
            }
            frame "Rub & Buzz Norm'd" {
              n231 = Build Array("Rub & Buzz Normalized" ("new element/subarray")) -> (w728:string[])
            }
            frame "Impulse Response" {
              w735 = u16 1 ("X data")
              n232 = Unbundle By Name(w731) -> ("Y data Time"=w732:u16, "dB ref Curve"=w734:dbl, "Y unit Curve"=w733:string)
              n233 = case shown="0, Default" w732 {
                tunnel: [w742 w746] -> w736
                tunnel: w734 -> [w744 _]
                tunnel: w733 -> [w743 w748]
                frame 0, Default {
                  n234 = Format Into String(format string="dB re %.p %s/s", w744, w743) -> (resulting string=w742:string)  [unwired: 2 in, 1 out]
                }
                frame 1 {
                  n235 = Format Into String(format string="%s/s", w748) -> (resulting string=w746:string)  [unwired: 2 in, 1 out]
                }
              }
              n236 = Bundle("X unit"="s", "X data"=w735, w736, "Y data Time"=w732, "Z unit"="", "X data"=w735) -> (w730:T12)  [unwired: 1 in]
              n237 = Build Array("Impulse Response" ("new element/subarray")) -> (w740:string[])
            }
            frame "Deconvolved Response" {
              w754 = u16 1 ("X data")
              n238 = Unbundle By Name(w749) -> ("Y data Time"=w751:u16, "dB ref Curve"=w753:dbl, "Y unit Curve"=w752:string)
              n239 = case shown="1" w751 {
                tunnel: [w761 w765] -> w755
                tunnel: w753 -> [w763 _]
                tunnel: w752 -> [w762 w767]
                frame 0, Default {
                  n240 = Format Into String(format string="dB re %.p %s/s", w763, w762) -> (resulting string=w761:string)  [unwired: 2 in, 1 out]
                }
                frame 1 {
                  n241 = Format Into String(format string="%s/s", w767) -> (resulting string=w765:string)  [unwired: 2 in, 1 out]
                }
              }
              n242 = Bundle("X unit"="s", "X data"=w754, w755, "Y data Time"=w751, "Z unit"="", "X data"=w754) -> (w750:T12)  [unwired: 1 in]
              n243 = Build Array("Deconvolved Response" ("new element/subarray")) -> (w759:string[])
            }
            frame Default {
            }
          }
        }
        frame "Multitone" {
          n244 = case shown="False" w776 {
            tunnel: w778 -> [w785 _]
            tunnel: w777 -> [w784 _]
            tunnel: [w783 "Impedence" ("new element/subarray")] -> w775
            tunnel: [w782 TRUE ("Result")] -> w773
            tunnel: [w781 T3 {"display X"=TRUE, "display Y"=TRUE, "display Z"=TRUE}] -> w772
            tunnel: w771 -> [w780 _]
            tunnel: [w779 _] -> w770
            frame False {
              n245 = case shown="\"Complex\"" w785 {
                tunnel: w784 -> [_ w794 w946]
                tunnel: ["" ("new element/subarray") w793 w945] -> w783
                tunnel: [FALSE ("Result") w792 w944] -> w782
                tunnel: [T3 {"display X"=FALSE, "display Y"=FALSE, "display Z"=FALSE} w791 w943] -> w781
                tunnel: w780 -> [_ w790 w942]
                tunnel: [_ w789 w941] -> w779
                frame "None", Default {
                }
                frame "Complex" {
                  n246 = case shown="\"Auto-Spectrum(Stimulus)\"" w794 {
                    tunnel: ["" ("new element/subarray") "Auto-Spectrum(Stimulus)" ("new element/subarray") "Auto-Spectrum(Response)" ("new element/subarray") "Frequency Response" ("new element/subarray") "Cross-Spectrum" ("new element/subarray") "Coherence" ("new element/subarray") "Non-Coherence" ("new element/subarray") "Signal-Noise Ratio" ("new element/subarray") "Coherent Power" ("new element/subarray") "Non-Coherent Power" ("new element/subarray") "Non-Coherent Distortion" ("new element/subarray")] -> w793
                    tunnel: [FALSE ("Result") TRUE ("Result") TRUE ("Result") TRUE ("Result") TRUE ("Result") TRUE ("Result") TRUE ("Result") TRUE ("Result") TRUE ("Result") TRUE ("Result") TRUE ("Result")] -> w792
                    tunnel: [T3 {"display X"=FALSE, "display Y"=FALSE, "display Z"=FALSE} T3 {"display X"=TRUE, "display Y"=TRUE, "display Z"=FALSE} T3 {"display X"=TRUE, "display Y"=TRUE, "display Z"=FALSE} T3 {"display X"=TRUE, "display Y"=TRUE, "display Z"=TRUE} T3 {"display X"=TRUE, "display Y"=TRUE, "display Z"=TRUE} T3 {"display X"=TRUE, "display Y"=TRUE, "display Z"=FALSE} T3 {"display X"=TRUE, "display Y"=TRUE, "display Z"=FALSE} T3 {"display X"=TRUE, "display Y"=TRUE, "display Z"=FALSE} T3 {"display X"=TRUE, "display Y"=TRUE, "display Z"=FALSE} T3 {"display X"=TRUE, "display Y"=TRUE, "display Z"=FALSE} T3 {"display X"=TRUE, "display Y"=TRUE, "display Z"=FALSE}] -> w791
                    tunnel: w790 -> [_ w798 w815 w833 w849 _ _ w888 w899 w918 _]
                    tunnel: [_ w799 w816 w832 w850 w873 w879 w890 w900 w917 w933] -> w789
                    frame "None", Default {
                    }
                    frame "Auto-Spectrum(Stimulus)" {
                      w803 = u16 1 ("X data")
                      n247 = Unbundle By Name(w798) -> ("Y data  Curve"=w800:u16, "dB ref Out"=w802:dbl, "Y unit Out"=w801:string)
                      n248 = case shown="0, Default" w800 {
                        tunnel: [w810 w811] -> w804
                        tunnel: w802 -> [_ w812]
                        tunnel: w801 -> [w810 w813]
                        frame 1 {
                        }
                        frame 0, Default {
                          n249 = Format Into String(format string="dB re %.p %s", w812, w813) -> (resulting string=w811:string)  [unwired: 2 in, 1 out]
                        }
                      }
                      n250 = Bundle("X unit"="Hz", "X data"=w803, "Y unit Out"=w804, "Y data  Curve"=w800, "Z unit"="", "X data"=w803) -> (w799:T10)  [unwired: 1 in]
                    }
                    frame "Auto-Spectrum(Response)" {
                      w820 = u16 1 ("X data")
                      n251 = Unbundle By Name(w815) -> ("Y data  Curve"=w817:u16, "dB ref In"=w819:dbl, "Y unit In"=w818:string)
                      n252 = case shown="0, Default" w817 {
                        tunnel: [w827 w828] -> w821
                        tunnel: w819 -> [_ w829]
                        tunnel: w818 -> [w827 w830]
                        frame 1 {
                        }
                        frame 0, Default {
                          n253 = Format Into String(format string="dB re %.p %s", w829, w830) -> (resulting string=w828:string)  [unwired: 2 in, 1 out]
                        }
                      }
                      n254 = Bundle("X unit"="Hz", "X data"=w820, "Y unit In"=w821, "Y data  Curve"=w817, "Z unit"="", "X data"=w820) -> (w816:T13)  [unwired: 1 in]
                    }
                    frame "Frequency Response" {
                      w837 = u16 1 ("X data")
                      n255 = Unbundle By Name(w833) -> ("Y data  Curve"=w834:u16, "dB ref Curve"=w836:dbl, "Y unit Curve"=w835:string)
                      n256 = case shown="0, Default" w834 {
                        tunnel: [w844 w845] -> w838
                        tunnel: w836 -> [_ w846]
                        tunnel: w835 -> [w844 w847]
                        frame 1 {
                        }
                        frame 0, Default {
                          n257 = Format Into String(format string="dB re %.p %s", w846, w847) -> (resulting string=w845:string)  [unwired: 2 in, 1 out]
                        }
                      }
                      n258 = Bundle("X unit"="Hz", "X data"=w837, "Y unit Curve"=w838, "Y data  Curve"=w834, "Z unit"="deg.", "X data"=w837) -> (w832:T8)  [unwired: 1 in]
                    }
                    frame "Cross-Spectrum" {
                      w855 = u16 1 ("X data")
                      n259 = Unbundle By Name(w849) -> ("Y data  Curve"=w858:u16, "dB ref In"=w856:dbl, "Y unit Out"=w857:string, "Y unit In"=w851:string)
                      n260 = case shown="1" w858 {
                        tunnel: [w864 w867] -> w854
                        tunnel: w856 -> [w865 _]
                        tunnel: w857 -> [w863 w869]
                        tunnel: w851 -> [w862 w868]
                        frame 0, Default {
                          n261 = Format Into String(format string="dB re %.p Sqrt(%s,%s)", w865, w863, w862) -> (resulting string=w864:string)  [unwired: 2 in, 1 out]
                        }
                        frame 1 {
                          n262 = Format Into String(format string="Sqrt(%s,%s)", w869, w868) -> (resulting string=w867:string)  [unwired: 2 in, 1 out]
                        }
                      }
                      n263 = Bundle("X unit"="Hz", "X data"=w855, w854, "Y data  Curve"=w858, "Z unit"="deg.", "X data"=w855) -> (w850:T9)  [unwired: 1 in]
                    }
                    frame "Coherence" {
                      w871 = u16 1 ("X data")
                      n264 = Bundle("X unit"="Hz", "X data"=w871, "X unit"="%", "X data"=w871, "Z unit"="", "X data"=w871) -> (w873:T11)  [unwired: 1 in]
                    }
                    frame "Non-Coherence" {
                      w880 = u16 1 ("X data")
                      n265 = Bundle("X unit"="Hz", "X data"=w880, "X unit"="%", "X data"=w880, "Z unit"="", "X data"=w880) -> (w879:T11)  [unwired: 1 in]
                    }
                    frame "Signal-Noise Ratio" {
                      w891 = u16 1 ("X data")
                      n266 = Unbundle By Name(w888) -> ("Y data  Curve"=w889:u16)
                      n267 = case shown="0, Default" w889 {
                        tunnel: ["dB re 1" ("X unit") "" ("Z unit")] -> w887
                        frame 0, Default {
                        }
                        frame 1 {
                        }
                      }
                      n268 = Bundle("X unit"="Hz", "X data"=w891, "Z unit"=w887, "X data"=w891, "Z unit"="", "X data"=w891) -> (w890:T14)  [unwired: 1 in]
                    }
                    frame "Coherent Power" {
                      w904 = u16 1 ("X data")
                      n269 = Unbundle By Name(w899) -> ("Y data  Curve"=w901:u16, "dB ref In"=w903:dbl, "Y unit In"=w902:string)
                      n270 = case shown="0, Default" w901 {
                        tunnel: [w911 w912] -> w905
                        tunnel: w903 -> [_ w913]
                        tunnel: w902 -> [w911 w914]
                        frame 1 {
                        }
                        frame 0, Default {
                          n271 = Format Into String(format string="dB re %.p %s", w913, w914) -> (resulting string=w912:string)  [unwired: 2 in, 1 out]
                        }
                      }
                      n272 = Bundle("X unit"="Hz", "X data"=w904, "Y unit In"=w905, "Y data  Curve"=w901, "Z unit"="", "X data"=w904) -> (w900:T13)  [unwired: 1 in]
                    }
                    frame "Non-Coherent Power" {
                      w922 = u16 1 ("X data")
                      n273 = Unbundle By Name(w918) -> ("Y data  Curve"=w919:u16, "dB ref In"=w921:dbl, "Y unit In"=w920:string)
                      n274 = case shown="0, Default" w919 {
                        tunnel: [w928 w929] -> w923
                        tunnel: w921 -> [_ w930]
                        tunnel: w920 -> [w928 w931]
                        frame 1 {
                        }
                        frame 0, Default {
                          n275 = Format Into String(format string="dB re %.p %s", w930, w931) -> (resulting string=w929:string)  [unwired: 2 in, 1 out]
                        }
                      }
                      n276 = Bundle("X unit"="Hz", "X data"=w922, "Y unit In"=w923, "Y data  Curve"=w919, "Z unit"="", "X data"=w922) -> (w917:T13)  [unwired: 1 in]
                    }
                    frame "Non-Coherent Distortion" {
                      w934 = u16 1 ("X data")
                      n277 = Bundle("X unit"="Hz", "X data"=w934, "X unit"="%", "X data"=w934, "Z unit"="", "X data"=w934) -> (w933:T11)  [unwired: 1 in]
                    }
                  }
                }
                frame "Power" {
                  n278 = case shown="\"Frequency Response\"" w946 {
                    tunnel: ["" ("new element/subarray") "Auto-Spectrum(Stimulus)" ("new element/subarray") "Auto-Spectrum(Response)" ("new element/subarray") "Frequency Response" ("new element/subarray")] -> w945
                    tunnel: [FALSE ("Result") TRUE ("Result") TRUE ("Result") TRUE ("Result")] -> w944
                    tunnel: [T3 {"display X"=FALSE, "display Y"=FALSE, "display Z"=FALSE} T3 {"display X"=TRUE, "display Y"=TRUE, "display Z"=FALSE} T3 {"display X"=TRUE, "display Y"=TRUE, "display Z"=FALSE} T3 {"display X"=TRUE, "display Y"=TRUE, "display Z"=TRUE}] -> w943
                    tunnel: w942 -> [_ w951 w968 w985]
                    tunnel: [_ w950 w967 w984] -> w941
                    frame "None", Default {
                    }
                    frame "Auto-Spectrum(Stimulus)" {
                      w955 = u16 1 ("X data")
                      n279 = Unbundle By Name(w951) -> ("Y data  Curve"=w958:u16, "dB ref Out"=w956:dbl, "Y unit Out"=w957:string)
                      n280 = case shown="0, Default" w958 {
                        tunnel: [w962 w963] -> w954
                        tunnel: w956 -> [_ w964]
                        tunnel: w957 -> [w962 w965]
                        frame 1 {
                        }
                        frame 0, Default {
                          n281 = Format Into String(format string="dB re %.p %s", w964, w965) -> (resulting string=w963:string)  [unwired: 2 in, 1 out]
                        }
                      }
                      n282 = Bundle("X unit"="Hz", "X data"=w955, "Y unit Out"=w954, "Y data  Curve"=w958, "Z unit"="", "X data"=w955) -> (w950:T10)  [unwired: 1 in]
                    }
                    frame "Auto-Spectrum(Response)" {
                      w972 = u16 1 ("X data")
                      n283 = Unbundle By Name(w968) -> ("Y data  Curve"=w975:u16, "dB ref In"=w973:dbl, "Y unit In"=w974:string)
                      n284 = case shown="0, Default" w975 {
                        tunnel: [w979 w980] -> w971
                        tunnel: w973 -> [_ w981]
                        tunnel: w974 -> [w979 w982]
                        frame 1 {
                        }
                        frame 0, Default {
                          n285 = Format Into String(format string="dB re %.p %s", w981, w982) -> (resulting string=w980:string)  [unwired: 2 in, 1 out]
                        }
                      }
                      n286 = Bundle("X unit"="Hz", "X data"=w972, "Y unit In"=w971, "Y data  Curve"=w975, "Z unit"="", "X data"=w972) -> (w967:T13)  [unwired: 1 in]
                    }
                    frame "Frequency Response" {
                      w989 = u16 1 ("X data")
                      n287 = Unbundle By Name(w985) -> ("Y data  Curve"=w992:u16, "dB ref Curve"=w990:dbl, "Y unit Curve"=w991:string)
                      n288 = case shown="0, Default" w992 {
                        tunnel: [w996 w997] -> w988
                        tunnel: w990 -> [_ w998]
                        tunnel: w991 -> [w996 w999]
                        frame 1 {
                        }
                        frame 0, Default {
                          n289 = Format Into String(format string="dB re %.p %s", w998, w999) -> (resulting string=w997:string)  [unwired: 2 in, 1 out]
                        }
                      }
                      n290 = Bundle("X unit"="Hz", "X data"=w989, "Y unit Curve"=w988, "Y data  Curve"=w992, "Z unit"="deg.", "X data"=w989) -> (w984:T8)  [unwired: 1 in]
                    }
                  }
                }
              }
            }
            frame True {
            }
          }
          n291 = Build Array(w775) -> (w774:string[])
        }
        frame "Transfer Function" {
          n292 = case shown="False" w1010 {
            tunnel: w1012 -> [w1019 _]
            tunnel: w1011 -> [w1018 _]
            tunnel: [w1017 "Impedence" ("new element/subarray")] -> w1009
            tunnel: [w1016 TRUE ("Result")] -> w1007
            tunnel: [w1015 T3 {"display X"=FALSE, "display Y"=FALSE, "display Z"=FALSE}] -> w1006
            tunnel: [w1014 _] -> w1005
            tunnel: w1004 -> [w1013 _]
            frame False {
              n293 = case shown="\"Complex\"" w1018 {
                tunnel: w1019 -> [_ w1028 w1255]
                tunnel: ["" ("new element/subarray") w1027 w1254] -> w1017
                tunnel: [FALSE ("Result") w1026 w1253] -> w1016
                tunnel: [T3 {"display X"=FALSE, "display Y"=FALSE, "display Z"=FALSE} w1025 w1252] -> w1015
                tunnel: [_ w1024 w1250] -> w1014
                tunnel: w1013 -> [_ w1023 w1251]
                frame "None", Default {
                }
                frame "Complex" {
                  n294 = case shown="\"Coherence\"" w1028 {
                    tunnel: ["" ("new element/subarray") "Auto-Spectrum(Stimulus)" ("new element/subarray") "Auto-Spectrum(Response)" ("new element/subarray") "Frequency Response" ("new element/subarray") "Cross-Spectrum" ("new element/subarray") "Coherence" ("new element/subarray") "Non-Coherence" ("new element/subarray") "Signal-Noise Ratio" ("new element/subarray") "Coherent Power" ("new element/subarray") "Non-Coherent Power" ("new element/subarray") "Non-Coherent Distortion" ("new element/subarray") "Impulse Response" ("new element/subarray") "Auto-Correlation(Stimulus)" ("new element/subarray") "Auto-Correlation(Response)" ("new element/subarray") "Cross-Correlation" ("new element/subarray")] -> w1027
                    tunnel: [FALSE ("Result") TRUE ("Result") TRUE ("Result") TRUE ("Result") TRUE ("Result") TRUE ("Result") TRUE ("Result") TRUE ("Result") TRUE ("Result") TRUE ("Result") FALSE ("Result") TRUE ("Result") TRUE ("Result") TRUE ("Result") TRUE ("Result")] -> w1026
                    tunnel: [T3 {"display X"=FALSE, "display Y"=FALSE, "display Z"=FALSE} T3 {"display X"=TRUE, "display Y"=TRUE, "display Z"=FALSE} T3 {"display X"=TRUE, "display Y"=TRUE, "display Z"=FALSE} T3 {"display X"=TRUE, "display Y"=TRUE, "display Z"=TRUE} T3 {"display X"=TRUE, "display Y"=TRUE, "display Z"=TRUE} T3 {"display X"=TRUE, "display Y"=TRUE, "display Z"=FALSE} T3 {"display X"=TRUE, "display Y"=TRUE, "display Z"=FALSE} T3 {"display X"=TRUE, "display Y"=TRUE, "display Z"=FALSE} T3 {"display X"=TRUE, "display Y"=TRUE, "display Z"=FALSE} T3 {"display X"=TRUE, "display Y"=TRUE, "display Z"=FALSE} T3 {"display X"=TRUE, "display Y"=TRUE, "display Z"=FALSE} T3 {"display X"=TRUE, "display Y"=TRUE, "display Z"=FALSE} T3 {"display X"=TRUE, "display Y"=TRUE, "display Z"=FALSE} T3 {"display X"=TRUE, "display Y"=TRUE, "display Z"=FALSE} T3 {"display X"=TRUE, "display Y"=TRUE, "display Z"=FALSE}] -> w1025
                    tunnel: [_ w1032 w1049 w1066 w1084 w1105 w1113 w1124 w1133 w1151 w1167 w1177 w1194 w1212 w1230] -> w1024
                    tunnel: w1023 -> [_ w1033 w1050 w1067 w1083 _ _ w1123 w1134 w1150 _ w1176 w1195 w1211 w1229]
                    frame "None", Default {
                    }
                    frame "Auto-Spectrum(Stimulus)" {
                      w1037 = u16 1 ("X data")
                      n295 = Unbundle By Name(w1033) -> ("Y data  Curve"=w1040:u16, "dB ref Out"=w1038:dbl, "Y unit Out"=w1039:string)
                      n296 = case shown="0, Default" w1040 {
                        tunnel: [w1044 w1045] -> w1036
                        tunnel: w1038 -> [_ w1046]
                        tunnel: w1039 -> [w1044 w1047]
                        frame 1 {
                        }
                        frame 0, Default {
                          n297 = Format Into String(format string="dB re %.p %s", w1046, w1047) -> (resulting string=w1045:string)  [unwired: 2 in, 1 out]
                        }
                      }
                      n298 = Bundle("X unit"="Hz", "X data"=w1037, "Y unit Out"=w1036, "Y data  Curve"=w1040, "Z unit"="", "X data"=w1037) -> (w1032:T10)  [unwired: 1 in]
                    }
                    frame "Auto-Spectrum(Response)" {
                      w1054 = u16 1 ("X data")
                      n299 = Unbundle By Name(w1050) -> ("Y data  Curve"=w1057:u16, "dB ref In"=w1055:dbl, "Y unit In"=w1056:string)
                      n300 = case shown="0, Default" w1057 {
                        tunnel: [w1061 w1062] -> w1053
                        tunnel: w1055 -> [_ w1063]
                        tunnel: w1056 -> [w1061 w1064]
                        frame 1 {
                        }
                        frame 0, Default {
                          n301 = Format Into String(format string="dB re %.p %s", w1063, w1064) -> (resulting string=w1062:string)  [unwired: 2 in, 1 out]
                        }
                      }
                      n302 = Bundle("X unit"="Hz", "X data"=w1054, "Y unit In"=w1053, "Y data  Curve"=w1057, "Z unit"="", "X data"=w1054) -> (w1049:T13)  [unwired: 1 in]
                    }
                    frame "Frequency Response" {
                      w1071 = u16 1 ("X data")
                      n303 = Unbundle By Name(w1067) -> ("Y data  Curve"=w1074:u16, "dB ref Curve"=w1072:dbl, "Y unit Curve"=w1073:string)
                      n304 = case shown="0, Default" w1074 {
                        tunnel: [w1078 w1079] -> w1070
                        tunnel: w1072 -> [_ w1080]
                        tunnel: w1073 -> [w1078 w1081]
                        frame 1 {
                        }
                        frame 0, Default {
                          n305 = Format Into String(format string="dB re %.p %s", w1080, w1081) -> (resulting string=w1079:string)  [unwired: 2 in, 1 out]
                        }
                      }
                      n306 = Bundle("X unit"="Hz", "X data"=w1071, "Y unit Curve"=w1070, "Y data  Curve"=w1074, "Z unit"="deg.", "X data"=w1071) -> (w1066:T8)  [unwired: 1 in]
                    }
                    frame "Cross-Spectrum" {
                      w1088 = u16 1 ("X data")
                      n307 = Unbundle By Name(w1083) -> ("Y data  Curve"=w1085:u16, "dB ref In"=w1087:dbl, "Y unit Out"=w1086:string, "Y unit In"=w1092:string)
                      n308 = case shown="0, Default" w1085 {
                        tunnel: [w1098 w1101] -> w1089
                        tunnel: w1087 -> [w1099 _]
                        tunnel: w1086 -> [w1097 w1103]
                        tunnel: w1092 -> [w1096 w1102]
                        frame 0, Default {
                          n309 = Format Into String(format string="dB re %.p Sqrt(%s,%s)", w1099, w1097, w1096) -> (resulting string=w1098:string)  [unwired: 2 in, 1 out]
                        }
                        frame 1 {
                          n310 = Format Into String(format string="Sqrt(%s,%s)", w1103, w1102) -> (resulting string=w1101:string)  [unwired: 2 in, 1 out]
                        }
                      }
                      n311 = Bundle("X unit"="Hz", "X data"=w1088, w1089, "Y data  Curve"=w1085, "Z unit"="deg.", "X data"=w1088) -> (w1084:T9)  [unwired: 1 in]
                    }
                    frame "Coherence" {
                      w1109 = u16 1 ("X data")
                      n312 = Bundle("X unit"="Hz", "X data"=w1109, "X unit"="%", "X data"=w1109, "Z unit"="", "X data"=w1109) -> (w1105:T11)  [unwired: 1 in]
                    }
                    frame "Non-Coherence" {
                      w1117 = u16 1 ("X data")
                      n313 = Bundle("X unit"="Hz", "X data"=w1117, "X unit"="%", "X data"=w1117, "Z unit"="", "X data"=w1117) -> (w1113:T11)  [unwired: 1 in]
                    }
                    frame "Signal-Noise Ratio" {
                      w1127 = u16 1 ("X data")
                      n314 = Unbundle By Name(w1123) -> ("Y data  Curve"=w1122:u16)
                      n315 = case shown="1" w1122 {
                        tunnel: ["dB re 1" ("X unit") "" ("Z unit")] -> w1121
                        frame 0, Default {
                        }
                        frame 1 {
                        }
                      }
                      n316 = Bundle("X unit"="Hz", "X data"=w1127, "Z unit"=w1121, "X data"=w1127, "Z unit"="", "X data"=w1127) -> (w1124:T14)  [unwired: 1 in]
                    }
                    frame "Coherent Power" {
                      w1138 = u16 1 ("X data")
                      n317 = Unbundle By Name(w1134) -> ("Y data  Curve"=w1141:u16, "dB ref In"=w1139:dbl, "Y unit In"=w1140:string)
                      n318 = case shown="0, Default" w1141 {
                        tunnel: [w1145 w1146] -> w1137
                        tunnel: w1139 -> [_ w1147]
                        tunnel: w1140 -> [w1145 w1148]
                        frame 1 {
                        }
                        frame 0, Default {
                          n319 = Format Into String(format string="dB re %.p %s", w1147, w1148) -> (resulting string=w1146:string)  [unwired: 2 in, 1 out]
                        }
                      }
                      n320 = Bundle("X unit"="Hz", "X data"=w1138, "Y unit In"=w1137, "Y data  Curve"=w1141, "Z unit"="", "X data"=w1138) -> (w1133:T13)  [unwired: 1 in]
                    }
                    frame "Non-Coherent Power" {
                      w1154 = u16 1 ("X data")
                      n321 = Unbundle By Name(w1150) -> ("Y data  Curve"=w1157:u16, "dB ref In"=w1155:dbl, "Y unit In"=w1156:string)
                      n322 = case shown="0, Default" w1157 {
                        tunnel: [w1162 w1163] -> w1153
                        tunnel: w1155 -> [_ w1164]
                        tunnel: w1156 -> [w1162 w1165]
                        frame 1 {
                        }
                        frame 0, Default {
                          n323 = Format Into String(format string="dB re %.p %s", w1164, w1165) -> (resulting string=w1163:string)  [unwired: 2 in, 1 out]
                        }
                      }
                      n324 = Bundle("X unit"="Hz", "X data"=w1154, "Y unit In"=w1153, "Y data  Curve"=w1157, "Z unit"="", "X data"=w1154) -> (w1151:T13)  [unwired: 1 in]
                    }
                    frame "Non-Coherent Distortion" {
                      w1171 = u16 1 ("X data")
                      n325 = Bundle("X unit"="Hz", "X data"=w1171, "X unit"="%", "X data"=w1171, "Z unit"="", "X data"=w1171) -> (w1167:T11)  [unwired: 1 in]
                    }
                    frame "Impulse Response" {
                      w1180 = u16 1 ("X data")
                      n326 = Unbundle By Name(w1176) -> ("Y data Time"=w1175:u16, "dB ref Curve"=w1179:dbl, "Y unit Curve"=w1178:string)
                      n327 = case shown="1" w1175 {
                        tunnel: [w1187 w1191] -> w1181
                        tunnel: w1179 -> [w1189 _]
                        tunnel: w1178 -> [w1188 w1193]
                        frame 0, Default {
                          n328 = Format Into String(format string="dB re %.p %s/s", w1189, w1188) -> (resulting string=w1187:string)  [unwired: 2 in, 1 out]
                        }
                        frame 1 {
                          n329 = Format Into String(format string="%s/s", w1193) -> (resulting string=w1191:string)  [unwired: 2 in, 1 out]
                        }
                      }
                      n330 = Bundle("X unit"="s", "X data"=w1180, w1181, "Y data Time"=w1175, "Z unit"="", "X data"=w1180) -> (w1177:T12)  [unwired: 1 in]
                    }
                    frame "Auto-Correlation(Stimulus)" {
                      w1199 = u16 1 ("X data")
                      n331 = Unbundle By Name(w1195) -> ("Y data Time"=w1202:u16, "dB ref Out"=w1200:dbl, "Y unit Out"=w1201:string)
                      n332 = case shown="0, Default" w1202 {
                        tunnel: [w1206 w1210] -> w1198
                        tunnel: w1200 -> [w1208 _]
                        tunnel: w1201 -> [w1207 w1210]
                        frame 0, Default {
                          n333 = Format Into String(format string="dB re %.p %s", w1208, w1207) -> (resulting string=w1206:string)  [unwired: 2 in, 1 out]
                        }
                        frame 1 {
                        }
                      }
                      n334 = Bundle("X unit"="s", "X data"=w1199, "Y unit Out"=w1198, "Y data Time"=w1202, "Z unit"="", "X data"=w1199) -> (w1194:T15)  [unwired: 1 in]
                    }
                    frame "Auto-Correlation(Response)" {
                      w1216 = u16 1 ("X data")
                      n335 = Unbundle By Name(w1211) -> ("Y data Time"=w1219:u16, "dB ref In"=w1217:dbl, "Y unit In"=w1218:string)
                      n336 = case shown="0, Default" w1219 {
                        tunnel: [w1223 w1227] -> w1215
                        tunnel: w1217 -> [w1224 _]
                        tunnel: w1218 -> [w1225 w1227]
                        frame 0, Default {
                          n337 = Format Into String(format string="dB re %.p %s", w1224, w1225) -> (resulting string=w1223:string)  [unwired: 2 in, 1 out]
                        }
                        frame 1 {
                        }
                      }
                      n338 = Bundle("X unit"="s", "X data"=w1216, "Y unit In"=w1215, "Y data Time"=w1219, "Z unit"="", "X data"=w1216) -> (w1212:T16)  [unwired: 1 in]
                    }
                    frame "Cross-Correlation" {
                      w1234 = u16 1 ("X data")
                      n339 = Unbundle By Name(w1229) -> ("Y data Time"=w1237:u16, "dB ref Curve"=w1235:dbl, "Y unit Out"=w1236:string, "Y unit In"=w1228:string)
                      n340 = case shown="0, Default" w1237 {
                        tunnel: [w1243 w1246] -> w1233
                        tunnel: w1235 -> [w1244 _]
                        tunnel: w1236 -> [w1242 w1248]
                        tunnel: w1228 -> [w1241 w1247]
                        frame 0, Default {
                          n341 = Format Into String(format string="dB re %.p sqrt(%s,%s)", w1244, w1242, w1241) -> (resulting string=w1243:string)  [unwired: 2 in, 1 out]
                        }
                        frame 1 {
                          n342 = Format Into String(format string="%s,%s", w1248, w1247) -> (resulting string=w1246:string)  [unwired: 2 in, 1 out]
                        }
                      }
                      n343 = Bundle("X unit"="s", "X data"=w1234, w1233, "Y data Time"=w1237, "Z unit"="", "X data"=w1234) -> (w1230:T12)  [unwired: 1 in]
                    }
                  }
                }
                frame "Power" {
                  n344 = case shown="\"Auto-Spectrum(Response)\"" w1255 {
                    tunnel: ["" ("new element/subarray") "Auto-Spectrum(Stimulus)" ("new element/subarray") "Auto-Spectrum(Response)" ("new element/subarray") "Frequency Response" ("new element/subarray") "Auto-Correlation(Stimulus)" ("new element/subarray") "Auto-Correlation(Response)" ("new element/subarray")] -> w1254
                    tunnel: [FALSE ("Result") TRUE ("Result") TRUE ("Result") TRUE ("Result") TRUE ("Result") TRUE ("Result")] -> w1253
                    tunnel: [T3 {"display X"=FALSE, "display Y"=FALSE, "display Z"=FALSE} T3 {"display X"=TRUE, "display Y"=TRUE, "display Z"=FALSE} T3 {"display X"=TRUE, "display Y"=TRUE, "display Z"=FALSE} T3 {"display X"=TRUE, "display Y"=TRUE, "display Z"=TRUE} T3 {"display X"=TRUE, "display Y"=TRUE, "display Z"=FALSE} T3 {"display X"=TRUE, "display Y"=TRUE, "display Z"=FALSE}] -> w1252
                    tunnel: w1251 -> [_ w1260 w1277 w1294 w1311 w1328]
                    tunnel: [_ w1259 w1276 w1293 w1310 w1327] -> w1250
                    frame "None", Default {
                    }
                    frame "Auto-Spectrum(Stimulus)" {
                      w1264 = u16 1 ("X data")
                      n345 = Unbundle By Name(w1260) -> ("Y data  Curve"=w1267:u16, "dB ref Out"=w1265:dbl, "Y unit Out"=w1266:string)
                      n346 = case shown="0, Default" w1267 {
                        tunnel: [w1271 w1272] -> w1263
                        tunnel: w1265 -> [_ w1273]
                        tunnel: w1266 -> [w1271 w1274]
                        frame 1 {
                        }
                        frame 0, Default {
                          n347 = Format Into String(format string="dB re %.p %s", w1273, w1274) -> (resulting string=w1272:string)  [unwired: 2 in, 1 out]
                        }
                      }
                      n348 = Bundle("X unit"="Hz", "X data"=w1264, "Y unit Out"=w1263, "Y data  Curve"=w1267, "Z unit"="", "X data"=w1264) -> (w1259:T10)  [unwired: 1 in]
                    }
                    frame "Auto-Spectrum(Response)" {
                      w1281 = u16 1 ("X data")
                      n349 = Unbundle By Name(w1277) -> ("Y data  Curve"=w1284:u16, "dB ref In"=w1282:dbl, "Y unit In"=w1283:string)
                      n350 = case shown="0, Default" w1284 {
                        tunnel: [w1288 w1289] -> w1280
                        tunnel: w1282 -> [_ w1290]
                        tunnel: w1283 -> [w1288 w1291]
                        frame 1 {
                        }
                        frame 0, Default {
                          n351 = Format Into String(format string="dB re %.p %s", w1290, w1291) -> (resulting string=w1289:string)  [unwired: 2 in, 1 out]
                        }
                      }
                      n352 = Bundle("X unit"="Hz", "X data"=w1281, "Y unit In"=w1280, "Y data  Curve"=w1284, "Z unit"="", "X data"=w1281) -> (w1276:T13)  [unwired: 1 in]
                    }
                    frame "Frequency Response" {
                      w1298 = u16 1 ("X data")
                      n353 = Unbundle By Name(w1294) -> ("Y data  Curve"=w1301:u16, "dB ref Curve"=w1299:dbl, "Y unit Curve"=w1300:string)
                      n354 = case shown="0, Default" w1301 {
                        tunnel: [w1305 w1306] -> w1297
                        tunnel: w1299 -> [_ w1307]
                        tunnel: w1300 -> [w1305 w1308]
                        frame 1 {
                        }
                        frame 0, Default {
                          n355 = Format Into String(format string="dB re %.p %s", w1307, w1308) -> (resulting string=w1306:string)  [unwired: 2 in, 1 out]
                        }
                      }
                      n356 = Bundle("X unit"="Hz", "X data"=w1298, "Y unit Curve"=w1297, "Y data  Curve"=w1301, "Z unit"="deg.", "X data"=w1298) -> (w1293:T8)  [unwired: 1 in]
                    }
                    frame "Auto-Correlation(Stimulus)" {
                      w1315 = u16 1 ("X data")
                      n357 = Unbundle By Name(w1311) -> ("Y data Time"=w1318:u16, "dB ref Out"=w1316:dbl, "Y unit Out"=w1317:string)
                      n358 = case shown="0, Default" w1318 {
                        tunnel: [w1322 w1326] -> w1314
                        tunnel: w1316 -> [w1324 _]
                        tunnel: w1317 -> [w1323 w1326]
                        frame 0, Default {
                          n359 = Format Into String(format string="dB re %.p %s", w1324, w1323) -> (resulting string=w1322:string)  [unwired: 2 in, 1 out]
                        }
                        frame 1 {
                        }
                      }
                      n360 = Bundle("X unit"="s", "X data"=w1315, "Y unit Out"=w1314, "Y data Time"=w1318, "Z unit"="", "X data"=w1315) -> (w1310:T15)  [unwired: 1 in]
                    }
                    frame "Auto-Correlation(Response)" {
                      w1332 = u16 1 ("X data")
                      n361 = Unbundle By Name(w1328) -> ("Y data Time"=w1335:u16, "dB ref In"=w1333:dbl, "Y unit In"=w1334:string)
                      n362 = case shown="0, Default" w1335 {
                        tunnel: [w1339 w1343] -> w1331
                        tunnel: w1333 -> [w1340 _]
                        tunnel: w1334 -> [w1341 w1343]
                        frame 0, Default {
                          n363 = Format Into String(format string="dB re %.p %s", w1340, w1341) -> (resulting string=w1339:string)  [unwired: 2 in, 1 out]
                        }
                        frame 1 {
                        }
                      }
                      n364 = Bundle("X unit"="s", "X data"=w1332, "Y unit In"=w1331, "Y data Time"=w1335, "Z unit"="", "X data"=w1332) -> (w1327:T16)  [unwired: 1 in]
                    }
                  }
                }
              }
            }
            frame True {
            }
          }
          n365 = Build Array(w1009) -> (w1008:string[])
        }
        frame Default {
        }
      }
    }
    frame True {
      n366 = case shown="\"Auto Delay\"" w1352 {
        tunnel: [w1357 w1370 string[] ["Loose Particle Envelope", "Loose Particle Threshold", "Loose Particle Count"] ("LooseParticleArray") string[] [] ("LooseParticleArray")] -> w1353
        tunnel: [TRUE ("Result") TRUE ("Result") TRUE ("Result") FALSE ("Result")] -> w1354
        tunnel: [T3 {"display X"=TRUE, "display Y"=TRUE, "display Z"=TRUE} T3 {"display X"=FALSE, "display Y"=TRUE, "display Z"=FALSE} T3 {"display X"=FALSE, "display Y"=TRUE, "display Z"=FALSE} T3 {"display X"=TRUE, "display Y"=TRUE, "display Z"=TRUE}] -> w1351
        tunnel: [_ w1360 w1377 _] -> w1350
        tunnel: w1349 -> [_ w1359 w1378 _]
        frame "Auto Delay" {
          # "make in engine directly."
          n367 = Build Array("Record Delay" ("RecordDelay")) -> (w1357:string[])
        }
        frame "Time Envelop" {
          w1364 = u16 1 ("X data")
          n368 = Unbundle By Name(w1359) -> ("Y data Time"=w1361:u16, "dB ref In"=w1363:dbl, "Y unit In"=w1362:string)
          n369 = case shown="0, Default" w1361 {
            tunnel: [w1372 w1373] -> w1365
            tunnel: w1363 -> [_ w1374]
            tunnel: w1362 -> [w1372 w1375]
            frame 1 {
            }
            frame 0, Default {
              n370 = Format Into String(format string="dB re %.p %s", w1374, w1375) -> (resulting string=w1373:string)  [unwired: 2 in, 1 out]
            }
          }
          n371 = Build Array("Time Envelope" ("TimeEnvelop")) -> (w1370:string[])
          n372 = Bundle("X unit"="s", "X data"=w1364, "Y unit In"=w1365, "Y data Time"=w1361, "Z unit"="", "X data"=w1364) -> (w1360:T16)  [unwired: 1 in]
        }
        frame "Loose Particle" {
          w1382 = u16 1 ("X data")
          # "Loose Particle Count ===== # ????????????"
          # "when no custom, unit 1"
          n373 = Unbundle By Name(w1378) -> ("Y data  Curve"=w1385:u16, "dB ref Curve"=w1383:dbl, "Y unit Curve"=w1384:string)
          n374 = case shown="0, Default" w1385 {
            tunnel: [w1389 w1393] -> w1381
            tunnel: w1383 -> [w1390 _]
            tunnel: w1384 -> [w1391 w1393]
            frame 0, Default {
              n375 = Format Into String(format string="dB re %.p %s", w1390, w1391) -> (resulting string=w1389:string)  [unwired: 2 in, 1 out]
            }
            frame 1 {
            }
          }
          n376 = Bundle("X unit"="s", "X data"=w1382, "Y unit Curve"=w1381, "Y data  Curve"=w1385, "Z unit"="", "X data"=w1382) -> (w1377:T8)  [unwired: 1 in]
        }
        frame Default {
        }
      }
    }
  }
  "Result" <- w17
  "Display" <- w4
  "Unit Info Out" <- w2
  "Curves Name Out" <- w16
